vi "Start Mode.vi"(8 "error in (no error)":errorcluster, 11 "RSeries_CAM in":refnum<class "RSeries_CAM.lvclass">) -> (0 "error out":errorcluster, 2 "Success?":bool, 3 "RSeries_CAM out":refnum<class "RSeries_CAM.lvclass">)   [LabVIEW 2024, in "RSeries_CAM.lvlib" / "RSeries_CAM.lvclass"]
uses:
  RSeries_CAM.lvclass
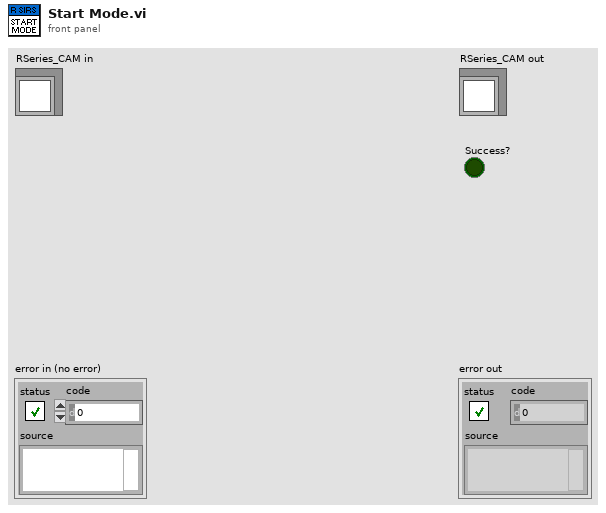
[diagram p1: front panel]
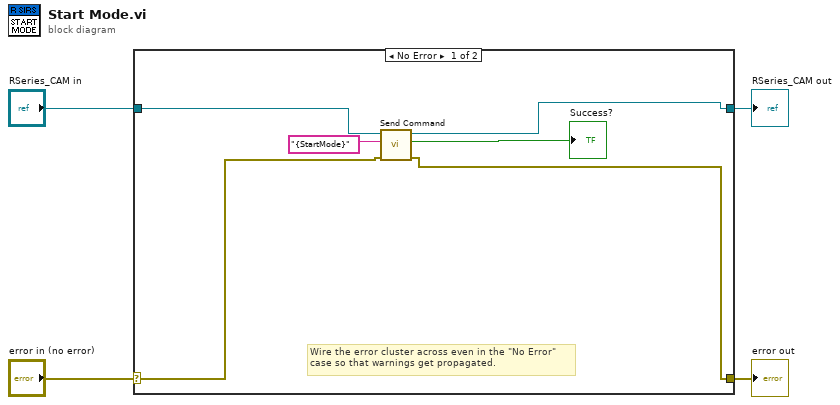
[diagram p0: block diagram]
diagram:
  n1 = case shown="No Error" "error in (no error)" {
    selector: "error in (no error)" -> [w6 w12]
    tunnel: [w5 w12] -> w3
    tunnel: [w9 w11] -> w1
    tunnel: "RSeries_CAM in" -> [w10 w11]
    frame No Error {
      # "Wire the error cluster across even in the \"No Error\"\ncase so that warnings get propagated."
      n2 = call "Send Command.vi"("error in (no error)"=w6, "Command"="{StartMode}", "RSeries_CAM in"=w10) -> ("error out"=w5:errorcluster, "Success?"=→"Success?":bool, "RSeries_CAM out"=w9:refnum<class "RSeries_CAM.lvclass">)  [unwired: 5 in, 1 out]
    }
    frame Error {
    }
  }
  "error out" <- w3
  "RSeries_CAM out" <- w1
